vi "Transmitter_Example_test.vi"() -> ()   [LabVIEW 2018]
uses:
  <vilib>/picture/picture.llb/imagedata.ctl
panel:
  out "new picture":picture
  out "image data":T1
  in  "path to BMP file":path
  in  "Modulation parameter":T2
  out "Bits length":i32
  out "Frame Duration":dbl format="%#_6p"
  out "Waveform Graph":cluster{"t0":dbl, "dt":dbl, "Y":dbl[]}(graph)
  in  "String":string="PENS"
  in  "USRP ControledParameters":T3={"active antenna"="TX1", "gain"=0.0, "carrier frequency"=915000000.0, "IQ rate"=1000000.0} {"IQ rate" format="%#_6p"; "carrier frequency" format="%#_6p"; "gain" format="%#_6f"}
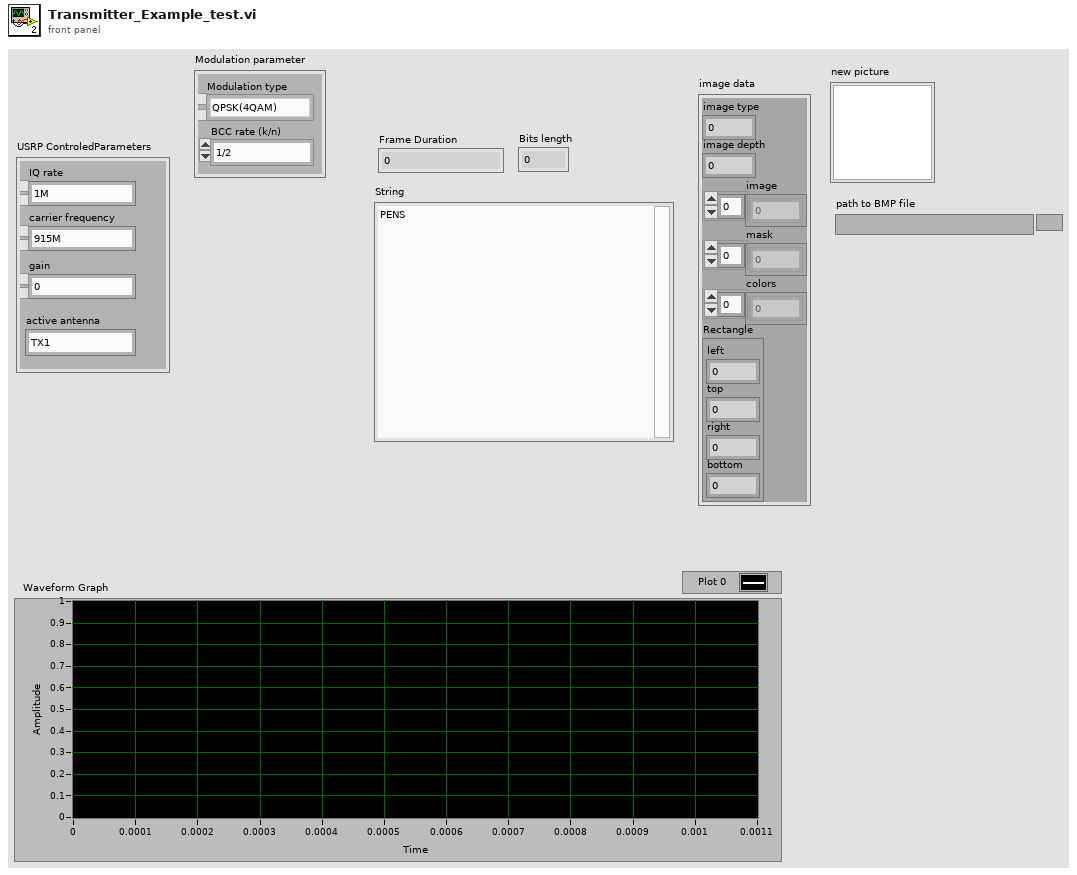
[diagram p1: front panel]
types:
  T1 = typedef "imagedata.ctl" = cluster{"image type":i32, "image depth":i32, "image":u8[], "mask":u8[], "colors":u32[], "Rectangle":cluster{"left":i16, "top":i16, "right":i16, "bottom":i16}}
  T2 = cluster{"Modulation type":enum16{"QPSK(4QAM)", "64QAM", "16QAM", "BPSK"}, "BCC rate (k/n)":enum16{"1/2", "2/3", "3/4"}}
  T3 = cluster{"active antenna":string, "gain":dbl, "carrier frequency":dbl, "IQ rate":dbl}
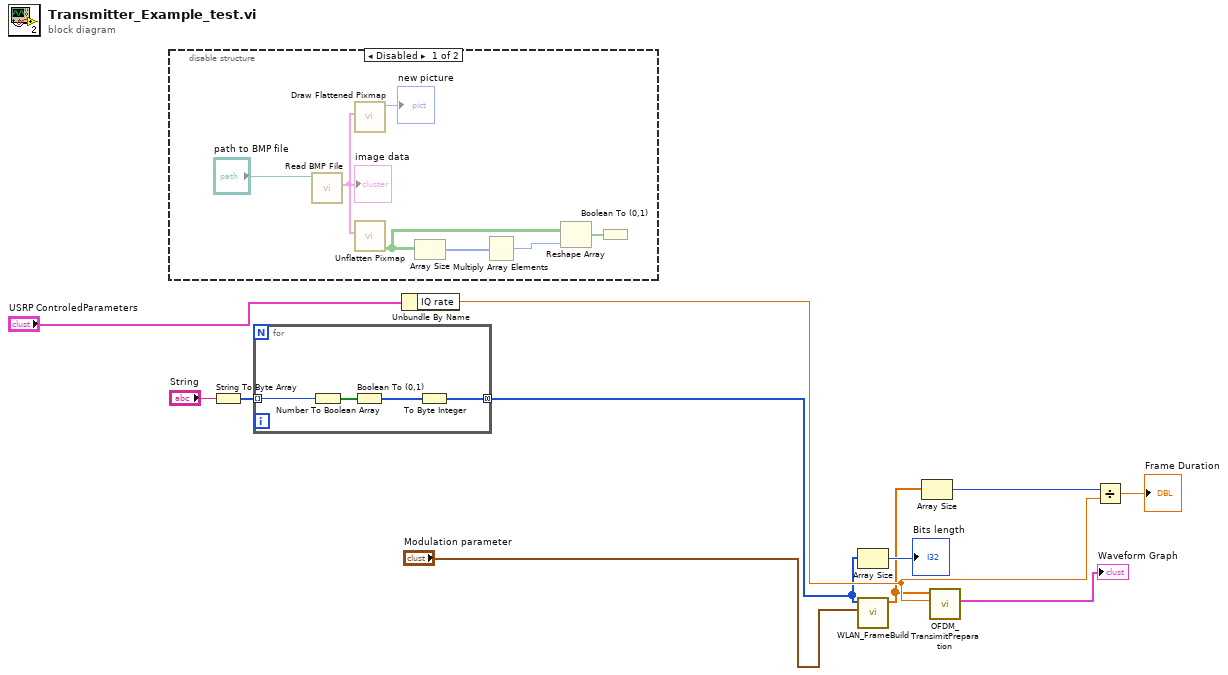
[diagram p0: block diagram]
diagram:
  n1 = disable-structure shown="Disabled" {
    frame Disabled {
      n2 = call <vilib>:"Read BMP File.vi"("path to BMP file"="path to BMP file") -> ("image data"=w16:T1)  [unwired: 8 in, 2 out]
      "image data" <- w16
      n3 = call <vilib>:"Draw Flattened Pixmap.vi"("image data"=w16) -> ("new picture"=→"new picture":picture)  [unwired: 8 in]
      n4 = call <vilib>:"Unflatten Pixmap.vi"("image data"=w16) -> ("1-bit pixmap"=w14:bool[][])  [unwired: 4 in, 6 out]
      n5 = Array Size(array=w14) -> (size(s)=w15:i32[])
      n6 = Multiply Array Elements(1:w15) -> (0:w13:i32)
      n7 = Reshape Array(w14, w13) -> (w12:bool[])
      n8 = Boolean To (0,1)(Boolean=w12) -> ()  [unwired: 1 out]
    }
    frame Enabled {
    }
  }
  n9 = String To Byte Array(string="String") -> (unsigned byte array=w8:u8[])
  n10 = for {
    tunnel: w8 -> [w22] mode=indexing
    tunnel: [w19] -> w6 mode=concatenating
    n11 = Number To Boolean Array(number=w22) -> (Boolean array=w21:bool[])
    n12 = Boolean To (0,1)(Boolean=w21) -> (0, 1=w20:i16[])
    n13 = To Byte Integer(number=w20) -> (8bit integer=w19:i8[])
  }
  n14 = Unbundle By Name("USRP ControledParameters") -> ("IQ rate"=w9:dbl)
  n15 = Array Size(array=w6) -> (size(s)=→"Bits length":i32)
  n16 = call "WLAN_FrameBuild.vi"("Modulation parameter"="Modulation parameter", "data in"=w6) -> ("output array"=w2:cdb[])  [unwired: 6 in, 3 out]
  n17 = Array Size(array=w2) -> (size(s)=w5:i32)
  n18 = call "OFDM_TransimitPreparation.vi"("IQ rate"=w9, "array"=w2) -> ("output cluster 2"=→"Waveform Graph":cluster{"t0":dbl, "dt":dbl, "Y":cdb[]})  [unwired: 8 in, 1 out]
  n19 = Divide(x=w5, y=w9) -> (x/y=→"Frame Duration":dbl)
